vi "Validate Checksum.vi"(10 "Response":string) -> (1 "Invalid Checksum?":bool, 2 "Remaining Response":string)   [LabVIEW 2018, in "Zaber A Series.lvlib"]
doc: "Expects a Zaber response string as an input. This VI inspects the response string to see if there is a checksum included. If not, then the same string is output and the boolean output is false. If there is a checksum, it is evaluated against the remainder of the response string. If the checksum is valid, the boolean output is false. If the checksum is not valid, the boolean output is true. Either way, the remainder of the response string (without the checksum) is output. For more information on checksums, see the web page here: https://www.zaber.com/protocol-manual#topic_checksums."
uses:
  Zaber A Series.lvlib
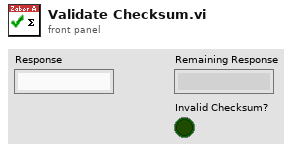
[diagram p1: front panel]
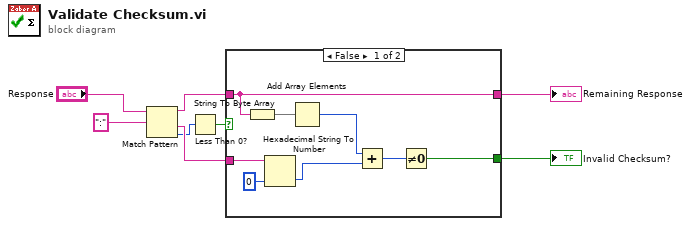
[diagram p0: block diagram]
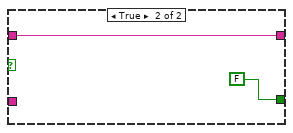
[diagram p2: hidden frame]
diagram:
  n1 = Match Pattern(string="Response", regular expression=":") -> (before substring=w5:string, after substring=w6:string, offset past match=w3:i32)  [unwired: 1 in, 1 out]
  n2 = Less Than 0?(x=w3) -> (x < 0?=w4:bool)
  n3 = case shown="False" w4 {
    tunnel: w6 -> [w16 _]
    tunnel: w5 -> [w13 w18]
    tunnel: [w13 w18] -> w1
    tunnel: [w9 FALSE] -> w2
    frame False {
      n4 = String To Byte Array(string=w13) -> (unsigned byte array=w12:u8[])
      n5 = Hexadecimal String To Number(string=w16, default (0uL)=i8 0 ("default (0 U32)")) -> (number=w15:i8)  [unwired: 1 in, 1 out]
      n6 = Add Array Elements(numeric array=w12) -> (sum=w11:u8)
      n7 = Add(x=w11, y=w15) -> (x+y=w10:u8)
      n8 = Not Equal To 0?(x=w10) -> (x != 0?=w9:bool)
    }
    frame True {
    }
  }
  "Invalid Checksum?" <- w2
  "Remaining Response" <- w1
